vi "Timer.vi"(7 "Action":enum16{"Reset", "Run", "Pause"}(ring), 8 "error in (no error)":errorcluster) -> (0 "error out":errorcluster, 3 "Time Elapsed [ms]":u32)   [LabVIEW 2020]
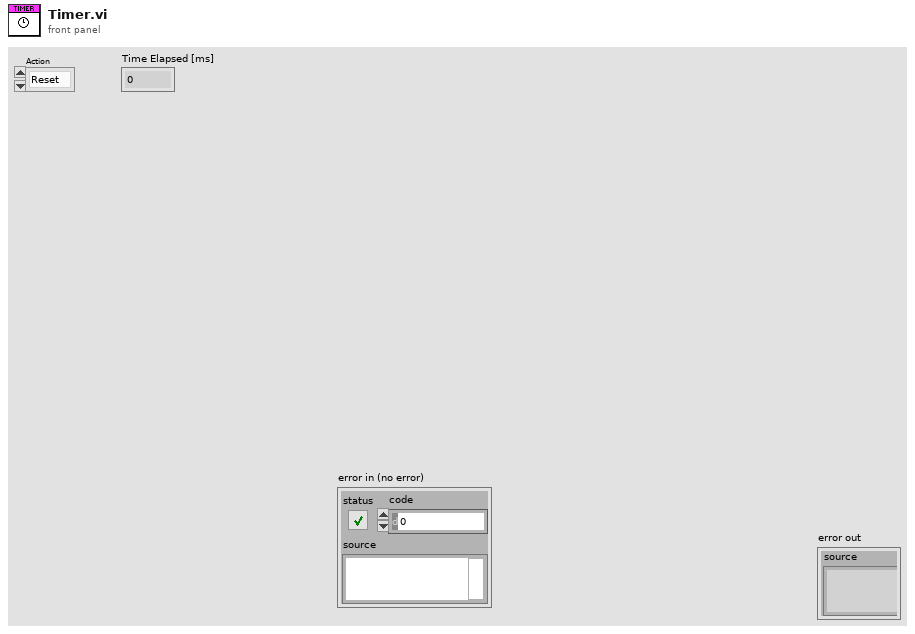
[diagram p1: front panel]
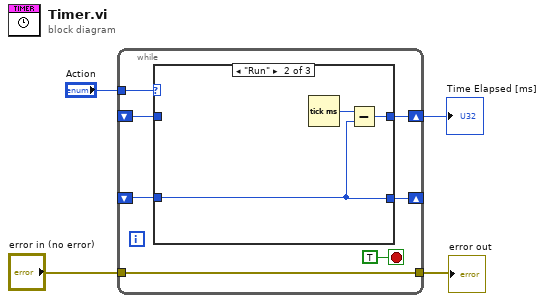
[diagram p0: block diagram]
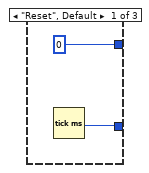
[diagram p2: hidden frame]
diagram:
  n1 = while {
    tunnel: "Action" -> [w10]
    shift-right: [w9] -> _
    shift-left: _ -> [w8]
    shift-right: [w7] -> w4
    shift-left: _ -> [w6]
    tunnel: "error in (no error)" -> [w5]
    tunnel: [w5] -> w1
    stop <- TRUE stop-if-true
    n2 = case shown="\"Run\"" w10 {
      tunnel: [w13 w15 w17] -> w9
      tunnel: w8 -> [_ w15 w17]
      tunnel: [u32 0 ("Time Elapsed [ms]") w14 w18] -> w7
      tunnel: w6 -> [_ _ w18]
      frame "Reset", Default {
        n3 = Tick Count (ms)() -> (millisecond timer value=w13:u32)
      }
      frame "Run" {
        n4 = Tick Count (ms)() -> (millisecond timer value=w16:u32)
        n5 = Subtract(x=w16, y=w15) -> (x-y=w14:u32)
      }
      frame "Pause" {
      }
    }
  }
  "Time Elapsed [ms]" <- w4
  "error out" <- w1
